vi "MPU_Stick_main.vi"() -> ()   [LabVIEW 2017]
uses:
  Controls/IMU_Accelerometer_Full_Scale_Values.ctl
  Controls/IMU_Accelerometer_Bandwidth.ctl
  Controls/IMU_Gyroscope_Full_Scale_Values.ctl
  Controls/IMU_Gyroscope_Bandwidth.ctl
  Controls/LED_config.ctl
  Controls/Motion_Detection_Threshold_Type.ctl
  Controls/MPU_Stick_Plotter_Parameters.ctl
  Controls/MPU_Stick_Globals.ctl
  Controls/IMU_Configuration_References.ctl
  Controls/MP_Comp_Filter_Constants_References.ctl
  Controls/MD_Threshold_References.ctl
  Controls/MD_Type_References.ctl
  Controls/LED_Configuration_References.ctl
  Controls/Primary_References.ctl
  Controls/MPU_Stick_Queues.ctl
  Controls/MPU_Stick_Queue_Element.ctl
  Controls/MPU_Stick_Queue_Commands.ctl
  Classes/ADCP.lvclass
panel:
  in  "Tab Control":enum32{"Configurations", "Data and plot"}(tab)
  in  "Save all config.":bool
  in  "Write all config.":bool
  in  "Read all config.":bool
  in  "Set pitch filter constant":bool
  in  "Get pitch filter constant":bool
  in  "Set roll filter constant":bool
  in  "Get roll filter constant":bool
  in  "Pitch filter constant":dbl
  in  "Roll filter constant":dbl
  in  "Get all Motion detection threshold configurations":bool
  in  "Set all Motion detection threshold configurations":bool
  in  "Set yaw threshold (upper)":bool
  in  "Get yaw threshold (upper)":bool
  in  "Set yaw threshold (lower)":bool
  in  "Get yaw threshold (lower)":bool
  in  "Set pitch threshold (upper)":bool
  in  "Get pitch threshold (upper)":bool
  in  "Set pitch threshold (lower)":bool
  in  "Get pitch threshold (lower)":bool
  in  "Set roll threshold (upper)":bool
  in  "Get roll threshold (upper)":bool
  in  "Set roll threshold (lower)":bool
  in  "Get roll threshold (lower)":bool
  in  "Yaw threshold (U)":dbl
  in  "Yaw threshold (L)":dbl
  in  "Pitch threshold (U)":dbl
  in  "Pitch. threshold (L)":dbl
  in  "Roll threshold (U)":dbl
  in  "Roll threshold (L)":dbl
  in  "Set Z gyro threshold (upper)":bool
  in  "Get Z gyro threshold (upper)":bool
  in  "Set Z gyro threshold (lower)":bool
  in  "Get Z gyro threshold (lower)":bool
  in  "Set Y gyro threshold (upper)":bool
  in  "Get Y gyro threshold (upper)":bool
  in  "Set Y gyro threshold (lower)":bool
  in  "Get Y gyro threshold (lower)":bool
  in  "Set X gyro threshold (upper)":bool
  in  "Get X gyro threshold (upper)":bool
  in  "Set X gyro threshold (lower)":bool
  in  "Get X gyro threshold (lower)":bool
  in  "Z gyro. threshold (U)":dbl
  in  "Z gyro. threshold (L)":dbl
  in  "Y gyro. threshold (U)":dbl
  in  "Y gyro. threshold (L)":dbl
  in  "X gyro. threshold (U)":dbl
  in  "X gyro. threshold (L)":dbl
  in  "Set Z accel threshold (upper)":bool
  in  "Get Z accel threshold (upper)":bool
  in  "Set Z accel threshold (lower)":bool
  in  "Get Z accel threshold (lower)":bool
  in  "Set Y accel threshold (upper)":bool
  in  "Get Y accel threshold (upper)":bool
  in  "Set Y accel threshold (lower)":bool
  in  "Get Y accel threshold (lower)":bool
  in  "Set X accel threshold (upper)":bool
  in  "Get X accel threshold (upper)":bool
  in  "Set X accel threshold (lower)":bool
  in  "Get X accel threshold (lower)":bool
  in  "Z accel. threshold (U)":dbl
  in  "Z accel. threshold (L)":dbl
  in  "Y accel. threshold (U)":dbl
  in  "Y accel. threshold (L)":dbl
  in  "X accel. threshold (U)":dbl
  in  "X accel. threshold (L)":dbl
  in  "Set all Motion detection type configurations":bool
  in  "Get all Motion detection type configurations":bool
  in  "Set yaw threshold type":bool
  in  "Get yaw threshold type":bool
  in  "Set pitch threshold type":bool
  in  "Get pitch threshold type":bool
  in  "Set roll threshold type":bool
  in  "Get roll threshold type":bool
  in  "Set Z gyroscope threshold type":bool
  in  "Get Z gyroscope threshold type":bool
  in  "Set Y gyroscope threshold type":bool
  in  "Get Y gyroscope threshold type":bool
  in  "Set X gyroscope threshold type":bool
  in  "Get X gyroscope threshold type":bool
  in  "Set Z accel threshold type":bool
  in  "Get Z accel threshold type":bool
  in  "Set Y accel threshold type":bool
  in  "Get Y accel threshold type":bool
  in  "Yaw threshold type":T1
  in  "Pitch threshold type":T1
  in  "Roll threshold type":T1
  in  "Z gyro threshold type":T1
  in  "Y gyro threshold type":T1
  in  "X gyro threshold type":T1
  in  "Z accel threshold type":T1
  in  "Y accel threshold type":T1
  in  "IMU Accelerometer F.S. value":T2
  in  "IMU Accelerometer bandwidth":T3
  in  "IMU Gyroscope F.S. value":T4
  in  "IMU Gyroscope bandwidth":T5
  in  "Calibration interval (ms)":u16
  in  "Calibration point count":u16
  in  "Sampling frequency (Hz)":u16
  in  "Set Accelerometer F.S. Value":bool
  in  "Get Accelerometer F.S. Value":bool
  in  "Set Accelerometer bandwidth":bool
  in  "Get Accelerometer bandwidth":bool
  in  "Set Gyroscope F.S. Value":bool
  in  "Get Gyroscope F.S. Value":bool
  in  "Set Gyroscope bandwidth":bool
  in  "Get Gyroscope bandwidth":bool
  in  "Set calibration interval":bool
  in  "Get calibration interval":bool
  in  "Set calibration point count":bool
  in  "Get calibration point count":bool
  in  "Set sampling frequency":bool
  in  "Get sampling frequency":bool
  in  "Set all IMU configurations":bool
  in  "Get all IMU configurations":bool
  in  "COM Port":refnum<visa-resource-name>="COM13"
  in  "Baud Rate":u32=38400
  in  "Connect Device":bool
  in  "LED1 Configuration":T6
  in  "LED2 Configuration":T6
  in  "LED3 Configuration":T6
  in  "Set LED1 configuration":bool
  in  "Get LED1 configuration":bool
  in  "Set LED2 configuration":bool
  in  "Get LED2 configuration":bool
  in  "Set LED3 configuration":bool
  in  "Get LED3 configuration":bool
  in  "Set all LED configurations":bool
  in  "Get all LED configurations":bool
  in  "X accel threshold type":T1
  in  "Set X accel threshold type":bool
  in  "Get X accel threshold type":bool
  out "Progress Bar":u8(slide) caption="No operation" scale=0.0..100.0
  out "Parameter name":string
  out "Plot time (ms)":dbl
  out "Plot value":dbl
  in  "Get Range & Offset":bool
  in  "Set Range & Offset":bool
  in  "Offset":dbl min=-100000.0 max=100000.0 step=0.1
  in  "Range":dbl min=0.0 max=100000.0 step=0.1
  in  "Exit Application":bool
  in  "Time (ms)":dbl
  in  "Value (Units)":dbl
  in  "Graph / 3D view tab control":enum32{"3D View", "Graph"}(tab)=enum."Graph"
  out "3D View Image":refnum<vi>(3d-picture)
  out "Plot":cluster{"Values":dbl[], "Time (ms)":dbl[]}[](graph)
  in  "MP Reset":bool
  in  "Calibrate IMU":bool
  out "Plot Parameter List":string[](array[string])
  in  "Remove Parameter from Plot":bool
  in  "Add Parameter to Plot":bool
  in  "Parameter to monitor":T7
  out "Yaw MD O/P":bool
  out "Pitch MD O/P":bool
  out "Roll MD O/P":bool
  out "Z gyro MD O/P":bool
  out "Y gyro MD O/P":bool
  out "X gyro MD O/P":bool
  out "Z accel MD O/P":bool
  out "Y accel MD O/P":bool
  out "X accel MD O/P":bool
  out "Roll angle (filter) (degrees)":dbl
  out "Pitch angle (filter) (degrees)":dbl
  out "Yaw angle (filter) (degrees)":dbl
  out "Roll angle (gyro) (degrees)":dbl
  out "Pitch angle (gyro) (degrees)":dbl
  out "Yaw angle (gyro) (degrees)":dbl
  out "Z accelerometer reading (G)":dbl
  out "Y accelerometer reading (G)":dbl
  out "X accelerometer reading (G)":dbl
  out "X gyroscope reading (DPS)":dbl
  out "Y gyroscope reading (DPS)":dbl
  out "Z gyroscope reading (DPS)":dbl
  out "Roll angle (accel) (degrees)":dbl
  out "Pitch angle (accel) (degrees)":dbl
  out "Yaw angle (accel) (degrees)":dbl
  # "LED CONFIGURATIONS"
  # "MOTION PROCESSING DETECTION CONFIGURATIONS"
  # "IMU CONFIGURATIONS"
  # "COMPLEMENTARY FILTER CONSTANTS"
  # "MOTION PROCESSED THRESHOLD CONFIGURATIONS"
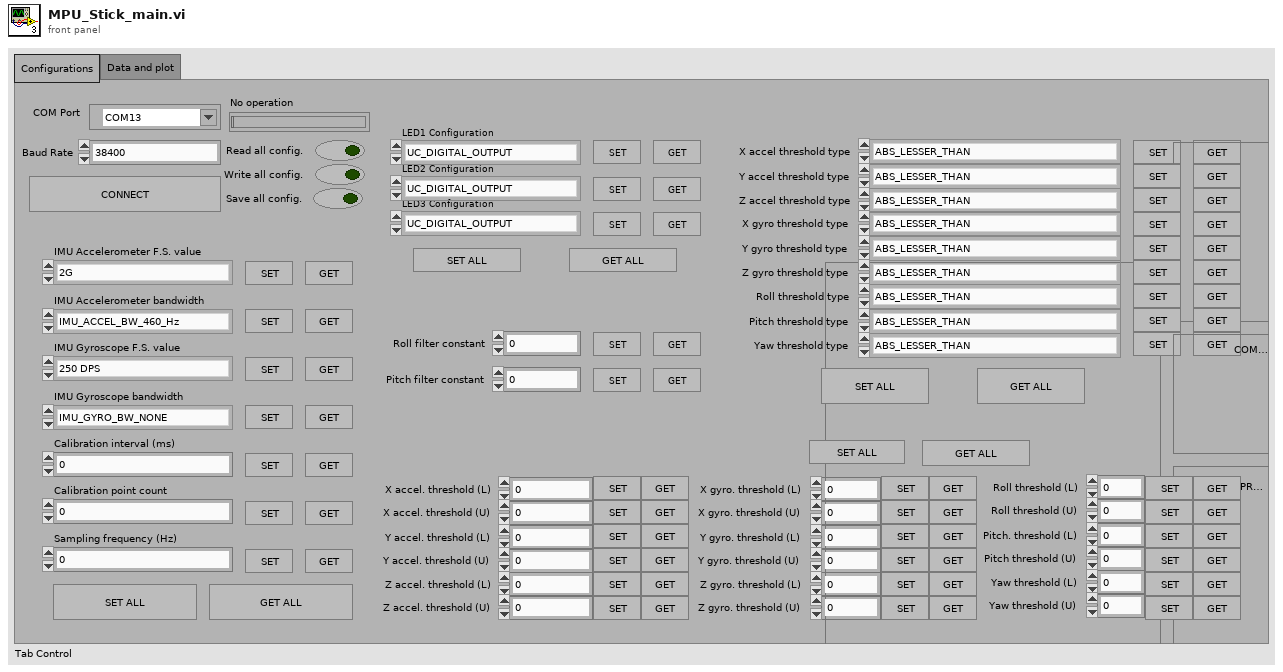
[diagram p1: front panel]
types:
  T1 = typedef "Motion_Detection_Threshold_Type.ctl" = enum16{"ABS_LESSER_THAN", "ABS_GREATER_THAN", "LESSER_THAN", "GREATER_THAN", "WINDOWED_MODE_WITHIN_BOUNDS", "WINDOWED_MODE_OUTSIDE_BOUNDS"}
  T2 = typedef "IMU_Accelerometer_Full_Scale_Values.ctl" = enum16{"2G", "4G", "8G", "16G"}
  T3 = typedef "IMU_Accelerometer_Bandwidth.ctl" = enum16{"IMU_ACCEL_BW_460_Hz", "IMU_ACCEL_BW_184_Hz", "IMU_ACCEL_BW_92_Hz", "IMU_ACCEL_BW_41_Hz", "IMU_ACCEL_BW_20_Hz", "IMU_ACCEL_BW_10_Hz", "IMU_ACCEL_BW_5_Hz"}
  T4 = typedef "IMU_Gyroscope_Full_Scale_Values.ctl" = enum16{"250 DPS", "500 DPS", "1000 DPS", "2000 DPS"}
  T5 = typedef "IMU_Gyroscope_Bandwidth.ctl" = enum16{"IMU_GYRO_BW_NONE", "IMU_GYRO_BW_184_Hz", "IMU_GYRO_BW_92_Hz", "IMU_GYRO_BW_41_Hz", "IMU_GYRO_BW_20_Hz", "IMU_GYRO_BW_10_Hz", "IMU_GYRO_BW_5_Hz"}
  T6 = typedef "LED_config.ctl" = enum16{"UC_DIGITAL_OUTPUT", "X_ACCEL_PWM", "Y_ACCEL_PWM", "Z_ACCEL_PWM", "X_ACCEL_MD_OUTPUT", "Y_ACCEL_MD_OUTPUT", "Z_ACCEL_MD_OUTPUT", "X_GYRO_PWM", "Y_GYRO_PWM", "Z_GYRO_PWM", "X_GYRO_MD_OUTPUT", "Y_GYRO_MD_OUTPUT", "Z_GYRO_MD_OUTPUT", "ROLL_PWM_OUTPUT", "PITCH_PWM_OUTPUT", "YAW_PWM_OUTPUT", "ROLL_MD_OUTPUT", "PITCH_MD_OUTPUT", "YAW_MD_OUTPUT", "UC_PWM_OUTPUT"}
  T7 = typedef "MPU_Stick_Plotter_Parameters.ctl" = enum16{"ACCEL_X", "ACCEL_Y", "ACCEL_Z", "GYRO_X", "GYRO_Y", "GYRO_Z", "ROLL_ACCEL", "ROLL_GYRO", "ROLL_COMP_FILTER", "PITCH_ACCEL", "PITCH_GYRO", "PITCH_COMP_FILTER", "YAW_ACCEL", "YAW_GYRO", "YAW_COMP_FILTER"}
  T8 = typedef "MPU_Stick_Globals.ctl" = cluster{"IMU_configuration_references":T9, "MP_Comp_Filter_Constants_References":T10, "MD_Threshold_References":T11, "MD_Type_References":T12, "LED_Configuration_References":T13, "Primary_references":T14, "MPU_Stick_Queues":T15, "ADCP":refnum<vi>}
  T9 = typedef "IMU_Configuration_References.ctl" = cluster{"Get all IMU configurations":refnum<vi>, "Set all IMU configurations":refnum<vi>, "Get sampling frequency":refnum<vi>, "Set sampling frequency":refnum<vi>, "Get calibration point count":refnum<vi>, "Set calibration point count":refnum<vi>, "Get calibration interval":refnum<vi>, "Set calibration interval":refnum<vi>, "Get Gyroscope bandwidth":refnum<vi>, "Set Gyroscope bandwidth":refnum<vi>, "Get Gyroscope F.S. Value":refnum<vi>, "Set Gyroscope F.S. Value":refnum<vi>, "Get Accelerometer bandwidth":refnum<vi>, "Set Accelerometer bandwidth":refnum<vi>, "Get Accelerometer F.S. Value":refnum<vi>, "Set Accelerometer F.S. Value":refnum<vi>, "Sampling frequency (Hz)":refnum<vi>, "Calibration point count":refnum<vi>, "Calibration interval (ms)":refnum<vi>, "IMU Gyroscope bandwidth":refnum<vi>, "IMU Gyroscope F.S. value":refnum<vi>, "IMU Accelerometer bandwidth":refnum<vi>, "IMU Accelerometer F.S. value":refnum<vi>}
  T10 = typedef "MP_Comp_Filter_Constants_References.ctl" = cluster{"Set pitch filter constant":refnum<vi>, "Get pitch filter constant":refnum<vi>, "Set roll filter constant":refnum<vi>, "Get roll filter constant":refnum<vi>, "Pitch filter constant":refnum<vi>, "Roll filter constant":refnum<vi>}
  T11 = typedef "MD_Threshold_References.ctl" = cluster{"Yaw threshold (U)":refnum<vi>, "Yaw threshold (L)":refnum<vi>, "Pitch threshold (U)":refnum<vi>, "Pitch. threshold (L)":refnum<vi>, "Roll threshold (U)":refnum<vi>, "Roll threshold (L)":refnum<vi>, "Z gyro. threshold (U)":refnum<vi>, "Z gyro. threshold (L)":refnum<vi>, "Y gyro. threshold (U)":refnum<vi>, "Y gyro. threshold (L)":refnum<vi>, "X gyro. threshold (U)":refnum<vi>, "X gyro. threshold (L)":refnum<vi>, "Z accel. threshold (U)":refnum<vi>, "Z accel. threshold (L)":refnum<vi>, "Y accel. threshold (U)":refnum<vi>, "Y accel. threshold (L)":refnum<vi>, "X accel. threshold (U)":refnum<vi>, "X accel. threshold (L)":refnum<vi>, "Set all Motion detection threshold configurations":refnum<vi>, "Get yaw threshold (upper)":refnum<vi>, "Get yaw threshold (lower)":refnum<vi>, "Get pitch threshold (upper)":refnum<vi>, "Get pitch threshold (lower)":refnum<vi>, "Get roll threshold (upper)":refnum<vi>, "Get roll threshold (lower)":refnum<vi>, "Get Z gyro threshold (upper)":refnum<vi>, "Get Z gyro threshold (lower)":refnum<vi>, "Get Y gyro threshold (upper)":refnum<vi>, "Get Y gyro threshold (lower)":refnum<vi>, "Get X gyro threshold (upper)":refnum<vi>, "Get X gyro threshold (lower)":refnum<vi>, "Get Z accel threshold (upper)":refnum<vi>, "Get Z accel threshold (lower)":refnum<vi>, "Get Y accel threshold (upper)":refnum<vi>, "Get Y accel threshold (lower)":refnum<vi>, "Get X accel threshold (upper)":refnum<vi>, "Get X accel threshold (lower)":refnum<vi>, "Get all Motion detection threshold configurations":refnum<vi>, "Set yaw threshold (upper)":refnum<vi>, "Set yaw threshold (lower)":refnum<vi>, "Set pitch threshold (upper)":refnum<vi>, "Set pitch threshold (lower)":refnum<vi>, "Set roll threshold (upper)":refnum<vi>, "Set roll threshold (lower)":refnum<vi>, "Set Z gyro threshold (upper)":refnum<vi>, "Set Z gyro threshold (lower)":refnum<vi>, "Set Y gyro threshold (upper)":refnum<vi>, "Set Y gyro threshold (lower)":refnum<vi>, "Set X gyro threshold (upper)":refnum<vi>, "Set X gyro threshold (lower)":refnum<vi>, "Set Z accel threshold (upper)":refnum<vi>, "Set Z accel threshold (lower)":refnum<vi>, "Set Y accel threshold (upper)":refnum<vi>, "Set Y accel threshold (lower)":refnum<vi>, "Set X accel threshold (upper)":refnum<vi>, "Set X accel threshold (lower)":refnum<vi>}
  T12 = typedef "MD_Type_References.ctl" = cluster{"Yaw threshold type":refnum<vi>, "Pitch threshold type":refnum<vi>, "Roll threshold type":refnum<vi>, "Z gyro threshold type":refnum<vi>, "Y gyro threshold type":refnum<vi>, "X gyro threshold type":refnum<vi>, "Z accel threshold type":refnum<vi>, "Y accel threshold type":refnum<vi>, "X accel threshold type":refnum<vi>, "Set all Motion detection type configurations":refnum<vi>, "Get all Motion detection type configurations":refnum<vi>, "Set yaw threshold type":refnum<vi>, "Get yaw threshold type":refnum<vi>, "Set pitch threshold type":refnum<vi>, "Get pitch threshold type":refnum<vi>, "Set roll threshold type":refnum<vi>, "Get roll threshold type":refnum<vi>, "Set Z gyroscope threshold type":refnum<vi>, "Get Z gyroscope threshold type":refnum<vi>, "Set Y gyroscope threshold type":refnum<vi>, "Get Y gyroscope threshold type":refnum<vi>, "Set X gyroscope threshold type":refnum<vi>, "Get X gyroscope threshold type":refnum<vi>, "Set Z accel threshold type":refnum<vi>, "Get Z accel threshold type":refnum<vi>, "Set Y accel threshold type":refnum<vi>, "Get Y accel threshold type":refnum<vi>, "Get X accel threshold type":refnum<vi>, "Set X accel threshold type":refnum<vi>}
  T13 = typedef "LED_Configuration_References.ctl" = cluster{"Get all LED configurations":refnum<vi>, "Set all LED configurations":refnum<vi>, "Get LED3 configuration":refnum<vi>, "Set LED3 configuration":refnum<vi>, "Get LED2 configuration":refnum<vi>, "Set LED2 configuration":refnum<vi>, "Get LED1 configuration":refnum<vi>, "Set LED1 configuration":refnum<vi>, "LED3 Configuration":refnum<vi>, "LED2 Configuration":refnum<vi>, "LED1 Configuration":refnum<vi>}
  T14 = typedef "Primary_References.ctl" = cluster{"3D View Image":refnum<vi>, "Plot":refnum<vi>, "Graph / 3D view tab control":refnum<vi>, "MP Reset":refnum<vi>, "Calibrate IMU":refnum<vi>, "Plot Parameter List":refnum<vi>, "Remove Parameter from Plot":refnum<vi>, "Add Parameter to Plot":refnum<vi>, "Parameter to monitor":refnum<vi>, "Yaw motion detection output":refnum<vi>, "Pitch motion detection output":refnum<vi>, "Roll motion detection output":refnum<vi>, "Z gyro motion detection output":refnum<vi>, "Y gyro motion detection output":refnum<vi>, "X gyro motion detection output":refnum<vi>, "Z accel motion detection output":refnum<vi>, "Y accel motion detection output":refnum<vi>, "X accel motion detection output":refnum<vi>, "Yaw angle (filter) (degrees)":refnum<vi>, "Pitch angle (filter) (degrees)":refnum<vi>, "Roll angle (filter) (degrees)":refnum<vi>, "Yaw angle (gyro) (degrees)":refnum<vi>, "Pitch angle (gyro) (degrees)":refnum<vi>, "Roll angle (gyro) (degrees)":refnum<vi>, "Yaw angle (accel) (degrees)":refnum<vi>, "Pitch angle (accel) (degrees)":refnum<vi>, "Roll angle (accel) (degrees)":refnum<vi>, "Z gyroscope reading (DPS)":refnum<vi>, "Y gyroscope reading (DPS)":refnum<vi>, "X gyroscope reading (DPS)":refnum<vi>, "Z accelerometer reading (G)":refnum<vi>, "Y accelerometer reading (G)":refnum<vi>, "X accelerometer reading (G)":refnum<vi>, "Save all config.":refnum<vi>, "Write all config.":refnum<vi>, "Read all config.":refnum<vi>, "Tab Control":refnum<vi>, "Baud Rate":refnum<vi>, "COM Port":refnum<vi>, "Time (ms)":refnum<vi>, "Value (Units)":refnum<vi>, "Exit Application":refnum<vi>, "Connect Device":refnum<vi>, "Progress Bar":refnum<vi>, "Get Range & Offset":refnum<vi>, "Range":refnum<vi>, "Offset":refnum<vi>, "Set Range & Offset":refnum<vi>, "Parameter name":refnum<vi>, "Plot time (ms)":refnum<vi>, "Plot value":refnum<vi>}
  T15 = typedef "MPU_Stick_Queues.ctl" = cluster{"UI Event Handler":refnum<queue>, "3D View Updater":refnum<queue>, "Plot Updater":refnum<queue>, "Serial Port Reader":refnum<queue>, "UI Indicators Updater":refnum<queue>}
diagram:
  n1 = control-ref of="This VI"() -> (w3:refnum<vi>)
  n2 = invoke class="VI" method="Default Vals.Reinit All"(reference=w3, error in=errorcluster {"status"=FALSE, "code"=0, "source"=""} ("error constant")) -> (error out=w4:errorcluster)  [unwired: 1 in, 2 out]
  n3 = flat-sequence {
    tunnel: w4 -> [w60]
    tunnel: [w60] -> w34
    tunnel: [w35] -> w29
    frame #0 {
      # "IMU Configuration Controls"
      n4 = control-ref of="Get Accelerometer F.S. Value"() -> (w44:refnum<vi>)
      n5 = control-ref of="Set Accelerometer F.S. Value"() -> (w43:refnum<vi>)
      n6 = control-ref of="Get all IMU configurations"() -> (w58:refnum<vi>)
      n7 = control-ref of="Get sampling frequency"() -> (w56:refnum<vi>)
      n8 = control-ref of="Set sampling frequency"() -> (w55:refnum<vi>)
      n9 = control-ref of="Set calibration point count"() -> (w53:refnum<vi>)
      n10 = control-ref of="Get calibration interval"() -> (w52:refnum<vi>)
      n11 = control-ref of="Set Gyroscope bandwidth"() -> (w49:refnum<vi>)
      n12 = control-ref of="Get Gyroscope F.S. Value"() -> (w48:refnum<vi>)
      n13 = control-ref of="Get Accelerometer bandwidth"() -> (w46:refnum<vi>)
      n14 = control-ref of="Set Accelerometer bandwidth"() -> (w45:refnum<vi>)
      n15 = control-ref of="Set all IMU configurations"() -> (w57:refnum<vi>)
      n16 = control-ref of="Get calibration point count"() -> (w54:refnum<vi>)
      n17 = control-ref of="Set calibration interval"() -> (w51:refnum<vi>)
      n18 = control-ref of="Get Gyroscope bandwidth"() -> (w50:refnum<vi>)
      n19 = control-ref of="Set Gyroscope F.S. Value"() -> (w47:refnum<vi>)
      n20 = control-ref of="Calibration interval (ms)"() -> (w40:refnum<vi>)
      n21 = control-ref of="Sampling frequency (Hz)"() -> (w42:refnum<vi>)
      n22 = control-ref of="Calibration point count"() -> (w41:refnum<vi>)
      n23 = control-ref of="IMU Gyroscope bandwidth"() -> (w39:refnum<vi>)
      n24 = control-ref of="IMU Gyroscope F.S. value"() -> (w38:refnum<vi>)
      n25 = control-ref of="IMU Accelerometer bandwidth"() -> (w37:refnum<vi>)
      n26 = control-ref of="IMU Accelerometer F.S. value"() -> (w36:refnum<vi>)
      n27 = Bundle By Name(cluster=T9 {"Get all IMU configurations"=refnum, "Set all IMU configurations"=refnum, "Get sampling frequency"=refnum, "Set sampling frequency"=refnum, "Get calibration point count"=refnum, "Set calibration point count"=refnum, "Get calibration interval"=refnum, "Set calibration interval"=refnum, "Get Gyroscope bandwidth"=refnum, "Set Gyroscope bandwidth"=refnum, "Get Gyroscope F.S. Value"=refnum, "Set Gyroscope F.S. Value"=refnum, "Get Accelerometer bandwidth"=refnum, "Set Accelerometer bandwidth"=refnum, "Get Accelerometer F.S. Value"=refnum, "Set Accelerometer F.S. Value"=refnum, "Sampling frequency (Hz)"=refnum, "Calibration point count"=refnum, "Calibration interval (ms)"=refnum, "IMU Gyroscope bandwidth"=refnum, "IMU Gyroscope F.S. value"=refnum, "IMU Accelerometer bandwidth"=refnum, "IMU Accelerometer F.S. value"=refnum} ("IMU configuration references"), "Get all IMU configurations"=w58, "Set all IMU configurations"=w57, "Get sampling frequency"=w56, "Set sampling frequency"=w55, "Get calibration point count"=w54, "Set calibration point count"=w53, "Get calibration interval"=w52, "Set calibration interval"=w51, "Get Gyroscope bandwidth"=w50, "Set Gyroscope bandwidth"=w49, "Get Gyroscope F.S. Value"=w48, "Set Gyroscope F.S. Value"=w47, "Get Accelerometer bandwidth"=w46, "Set Accelerometer bandwidth"=w45, "Get Accelerometer F.S. Value"=w44, "Set Accelerometer F.S. Value"=w43, "Sampling frequency (Hz)"=w42, "Calibration point count"=w41, "Calibration interval (ms)"=w40, "IMU Gyroscope bandwidth"=w39, "IMU Gyroscope F.S. value"=w38, "IMU Accelerometer bandwidth"=w37, "IMU Accelerometer F.S. value"=w36) -> (w35:T9)
    }
  }
  n28 = flat-sequence {
    tunnel: w34 -> [w115]
    tunnel: [w115] -> w33
    tunnel: w29 -> [w73]
    tunnel: [w73] -> w28
    tunnel: [w72] -> w24
    frame #0 {
      # "UI primary controls & indicators"
      n29 = control-ref of="MP Reset"() -> (w110:refnum<vi>)
      n30 = control-ref of="Graph / 3D view tab control"() -> (w111:refnum<vi>)
      n31 = control-ref of="Calibrate IMU"() -> (w109:refnum<vi>)
      n32 = control-ref of="3D View Image"() -> (w113:refnum<vi>)
      n33 = control-ref of="Plot"() -> (w112:refnum<vi>)
      n34 = control-ref of="X accel MD O/P"() -> (w96:refnum<vi>)
      n35 = control-ref of="Y accel MD O/P"() -> (w97:refnum<vi>)
      n36 = control-ref of="Plot Parameter List"() -> (w108:refnum<vi>)
      n37 = control-ref of="Remove Parameter from Plot"() -> (w107:refnum<vi>)
      n38 = control-ref of="Add Parameter to Plot"() -> (w106:refnum<vi>)
      n39 = control-ref of="Parameter to monitor"() -> (w105:refnum<vi>)
      n40 = control-ref of="X gyro MD O/P"() -> (w99:refnum<vi>)
      n41 = control-ref of="Z accel MD O/P"() -> (w98:refnum<vi>)
      n42 = control-ref of="Yaw angle (filter) (degrees)"() -> (w95:refnum<vi>)
      n43 = control-ref of="Yaw MD O/P"() -> (w104:refnum<vi>)
      n44 = control-ref of="Pitch MD O/P"() -> (w103:refnum<vi>)
      n45 = control-ref of="Roll MD O/P"() -> (w102:refnum<vi>)
      n46 = control-ref of="Z gyro MD O/P"() -> (w101:refnum<vi>)
      n47 = control-ref of="Y gyro MD O/P"() -> (w100:refnum<vi>)
      n48 = control-ref of="Pitch angle (filter) (degrees)"() -> (w94:refnum<vi>)
      n49 = control-ref of="COM Port"() -> (w74:refnum<vi>)
      n50 = control-ref of="Roll angle (filter) (degrees)"() -> (w93:refnum<vi>)
      n51 = control-ref of="Save all config."() -> (w80:refnum<vi>)
      n52 = control-ref of="Write all config."() -> (w79:refnum<vi>)
      n53 = control-ref of="Tab Control"() -> (w77:refnum<vi>)
      n54 = control-ref of="Connect Device"() -> (w76:refnum<vi>)
      n55 = control-ref of="Baud Rate"() -> (w75:refnum<vi>)
      n56 = control-ref of="Pitch angle (gyro) (degrees)"() -> (w91:refnum<vi>)
      n57 = control-ref of="X gyroscope reading (DPS)"() -> (w84:refnum<vi>)
      n58 = control-ref of="Read all config."() -> (w78:refnum<vi>)
      n59 = control-ref of="Yaw angle (gyro) (degrees)"() -> (w92:refnum<vi>)
      n60 = control-ref of="Roll angle (gyro) (degrees)"() -> (w90:refnum<vi>)
      n61 = control-ref of="Yaw angle (accel) (degrees)"() -> (w89:refnum<vi>)
      n62 = control-ref of="Roll angle (accel) (degrees)"() -> (w87:refnum<vi>)
      n63 = control-ref of="Z gyroscope reading (DPS)"() -> (w86:refnum<vi>)
      n64 = control-ref of="Y gyroscope reading (DPS)"() -> (w85:refnum<vi>)
      n65 = control-ref of="Time (ms)"() -> (w71:refnum<vi>)
      n66 = control-ref of="Value (Units)"() -> (w70:refnum<vi>)
      n67 = control-ref of="Exit Application"() -> (w69:refnum<vi>)
      n68 = control-ref of="Progress Bar"() -> (w68:refnum<vi>)
      n69 = control-ref of="Pitch angle (accel) (degrees)"() -> (w88:refnum<vi>)
      n70 = control-ref of="Z accelerometer reading (G)"() -> (w83:refnum<vi>)
      n71 = control-ref of="Y accelerometer reading (G)"() -> (w82:refnum<vi>)
      n72 = control-ref of="X accelerometer reading (G)"() -> (w81:refnum<vi>)
      n73 = control-ref of="Get Range & Offset"() -> (w67:refnum<vi>)
      n74 = control-ref of="Range"() -> (w66:refnum<vi>)
      n75 = control-ref of="Offset"() -> (w65:refnum<vi>)
      n76 = control-ref of="Set Range & Offset"() -> (w64:refnum<vi>)
      n77 = control-ref of="Parameter name"() -> (w63:refnum<vi>)
      n78 = control-ref of="Plot time (ms)"() -> (w62:refnum<vi>)
      n79 = control-ref of="Plot value"() -> (w61:refnum<vi>)
      n80 = Bundle By Name(cluster=T14 {"3D View Image"=refnum, "Plot"=refnum, "Graph / 3D view tab control"=refnum, "MP Reset"=refnum, "Calibrate IMU"=refnum, "Plot Parameter List"=refnum, "Remove Parameter from Plot"=refnum, "Add Parameter to Plot"=refnum, "Parameter to monitor"=refnum, "Yaw motion detection output"=refnum, "Pitch motion detection output"=refnum, "Roll motion detection output"=refnum, "Z gyro motion detection output"=refnum, "Y gyro motion detection output"=refnum, "X gyro motion detection output"=refnum, "Z accel motion detection output"=refnum, "Y accel motion detection output"=refnum, "X accel motion detection output"=refnum, "Yaw angle (filter) (degrees)"=refnum, "Pitch angle (filter) (degrees)"=refnum, "Roll angle (filter) (degrees)"=refnum, "Yaw angle (gyro) (degrees)"=refnum, "Pitch angle (gyro) (degrees)"=refnum, "Roll angle (gyro) (degrees)"=refnum, "Yaw angle (accel) (degrees)"=refnum, "Pitch angle (accel) (degrees)"=refnum, "Roll angle (accel) (degrees)"=refnum, "Z gyroscope reading (DPS)"=refnum, "Y gyroscope reading (DPS)"=refnum, "X gyroscope reading (DPS)"=refnum, "Z accelerometer reading (G)"=refnum, "Y accelerometer reading (G)"=refnum, "X accelerometer reading (G)"=refnum, "Save all config."=refnum, "Write all config."=refnum, "Read all config."=refnum, "Tab Control"=refnum, "Baud Rate"=refnum, "COM Port"=refnum, "Time (ms)"=refnum, "Value (Units)"=refnum, "Exit Application"=refnum, "Connect Device"=refnum, "Progress Bar"=refnum, "Get Range & Offset"=refnum, "Range"=refnum, "Offset"=refnum, "Set Range & Offset"=refnum, "Parameter name"=refnum, "Plot time (ms)"=refnum, "Plot value"=refnum}, "3D View Image"=w113, "Plot"=w112, "Graph / 3D view tab control"=w111, "MP Reset"=w110, "Calibrate IMU"=w109, "Plot Parameter List"=w108, "Remove Parameter from Plot"=w107, "Add Parameter to Plot"=w106, "Parameter to monitor"=w105, "Yaw motion detection output"=w104, "Pitch motion detection output"=w103, "Roll motion detection output"=w102, "Z gyro motion detection output"=w101, "Y gyro motion detection output"=w100, "X gyro motion detection output"=w99, "Z accel motion detection output"=w98, "Y accel motion detection output"=w97, "X accel motion detection output"=w96, "Yaw angle (filter) (degrees)"=w95, "Pitch angle (filter) (degrees)"=w94, "Roll angle (filter) (degrees)"=w93, "Yaw angle (gyro) (degrees)"=w92, "Pitch angle (gyro) (degrees)"=w91, "Roll angle (gyro) (degrees)"=w90, "Yaw angle (accel) (degrees)"=w89, "Pitch angle (accel) (degrees)"=w88, "Roll angle (accel) (degrees)"=w87, "Z gyroscope reading (DPS)"=w86, "Y gyroscope reading (DPS)"=w85, "X gyroscope reading (DPS)"=w84, "Z accelerometer reading (G)"=w83, "Y accelerometer reading (G)"=w82, "X accelerometer reading (G)"=w81, "Save all config."=w80, "Write all config."=w79, "Read all config."=w78, "Tab Control"=w77, "Connect Device"=w76, "Baud Rate"=w75, "COM Port"=w74, "Time (ms)"=w71, "Value (Units)"=w70, "Exit Application"=w69, "Progress Bar"=w68, "Get Range & Offset"=w67, "Range"=w66, "Offset"=w65, "Set Range & Offset"=w64, "Parameter name"=w63, "Plot time (ms)"=w62, "Plot value"=w61) -> (w72:T14)
    }
  }
  n81 = flat-sequence {
    tunnel: w33 -> [w131]
    tunnel: [w131] -> w32
    tunnel: w28 -> [w118]
    tunnel: [w118] -> w27
    tunnel: w24 -> [w117]
    tunnel: [w117] -> w23
    tunnel: [w116] -> w20
    frame #0 {
      # "LED configurations"
      n82 = control-ref of="Get all LED configurations"() -> (w129:refnum<vi>)
      n83 = control-ref of="Set all LED configurations"() -> (w128:refnum<vi>)
      n84 = control-ref of="Get LED3 configuration"() -> (w127:refnum<vi>)
      n85 = control-ref of="Set LED3 configuration"() -> (w126:refnum<vi>)
      n86 = control-ref of="Get LED2 configuration"() -> (w125:refnum<vi>)
      n87 = control-ref of="Set LED2 configuration"() -> (w124:refnum<vi>)
      n88 = control-ref of="Get LED1 configuration"() -> (w123:refnum<vi>)
      n89 = control-ref of="Set LED1 configuration"() -> (w122:refnum<vi>)
      n90 = control-ref of="LED3 Configuration"() -> (w121:refnum<vi>)
      n91 = control-ref of="LED2 Configuration"() -> (w120:refnum<vi>)
      n92 = control-ref of="LED1 Configuration"() -> (w119:refnum<vi>)
      n93 = Bundle By Name(cluster=T13 {"Get all LED configurations"=refnum, "Set all LED configurations"=refnum, "Get LED3 configuration"=refnum, "Set LED3 configuration"=refnum, "Get LED2 configuration"=refnum, "Set LED2 configuration"=refnum, "Get LED1 configuration"=refnum, "Set LED1 configuration"=refnum, "LED3 Configuration"=refnum, "LED2 Configuration"=refnum, "LED1 Configuration"=refnum}, "Get all LED configurations"=w129, "Set all LED configurations"=w128, "Get LED3 configuration"=w127, "Set LED3 configuration"=w126, "Get LED2 configuration"=w125, "Set LED2 configuration"=w124, "Get LED1 configuration"=w123, "Set LED1 configuration"=w122, "LED3 Configuration"=w121, "LED2 Configuration"=w120, "LED1 Configuration"=w119) -> (w116:T13)
    }
  }
  n94 = flat-sequence {
    tunnel: w32 -> [w167]
    tunnel: [w167] -> w31
    tunnel: w27 -> [w135]
    tunnel: [w135] -> w26
    tunnel: w23 -> [w134]
    tunnel: [w134] -> w22
    tunnel: w20 -> [w133]
    tunnel: [w133] -> w19
    tunnel: [w132] -> w17
    frame #0 {
      # "Motion detection threshold types"
      n95 = control-ref of="Yaw threshold type"() -> (w165:refnum<vi>)
      n96 = control-ref of="Pitch threshold type"() -> (w164:refnum<vi>)
      n97 = control-ref of="Roll threshold type"() -> (w163:refnum<vi>)
      n98 = control-ref of="Z gyro threshold type"() -> (w162:refnum<vi>)
      n99 = control-ref of="Y gyro threshold type"() -> (w161:refnum<vi>)
      n100 = control-ref of="X gyro threshold type"() -> (w160:refnum<vi>)
      n101 = control-ref of="Z accel threshold type"() -> (w159:refnum<vi>)
      n102 = control-ref of="Y accel threshold type"() -> (w158:refnum<vi>)
      n103 = control-ref of="X accel threshold type"() -> (w157:refnum<vi>)
      n104 = Bundle By Name(cluster=T12 {"Yaw threshold type"=refnum, "Pitch threshold type"=refnum, "Roll threshold type"=refnum, "Z gyro threshold type"=refnum, "Y gyro threshold type"=refnum, "X gyro threshold type"=refnum, "Z accel threshold type"=refnum, "Y accel threshold type"=refnum, "X accel threshold type"=refnum, "Set all Motion detection type configurations"=refnum, "Get all Motion detection type configurations"=refnum, "Set yaw threshold type"=refnum, "Get yaw threshold type"=refnum, "Set pitch threshold type"=refnum, "Get pitch threshold type"=refnum, "Set roll threshold type"=refnum, "Get roll threshold type"=refnum, "Set Z gyroscope threshold type"=refnum, "Get Z gyroscope threshold type"=refnum, "Set Y gyroscope threshold type"=refnum, "Get Y gyroscope threshold type"=refnum, "Set X gyroscope threshold type"=refnum, "Get X gyroscope threshold type"=refnum, "Set Z accel threshold type"=refnum, "Get Z accel threshold type"=refnum, "Set Y accel threshold type"=refnum, "Get Y accel threshold type"=refnum, "Get X accel threshold type"=refnum, "Set X accel threshold type"=refnum}, "Yaw threshold type"=w165, "Pitch threshold type"=w164, "Roll threshold type"=w163, "Z gyro threshold type"=w162, "Y gyro threshold type"=w161, "X gyro threshold type"=w160, "Z accel threshold type"=w159, "Y accel threshold type"=w158, "X accel threshold type"=w157) -> (w156:T12)
      n105 = control-ref of="Set all Motion detection type configurations"() -> (w155:refnum<vi>)
      n106 = control-ref of="Get all Motion detection type configurations"() -> (w154:refnum<vi>)
      n107 = control-ref of="Set yaw threshold type"() -> (w153:refnum<vi>)
      n108 = control-ref of="Get yaw threshold type"() -> (w152:refnum<vi>)
      n109 = control-ref of="Set pitch threshold type"() -> (w151:refnum<vi>)
      n110 = control-ref of="Get pitch threshold type"() -> (w150:refnum<vi>)
      n111 = control-ref of="Set roll threshold type"() -> (w149:refnum<vi>)
      n112 = control-ref of="Get roll threshold type"() -> (w148:refnum<vi>)
      n113 = control-ref of="Set Z gyroscope threshold type"() -> (w147:refnum<vi>)
      n114 = control-ref of="Get Z gyroscope threshold type"() -> (w146:refnum<vi>)
      n115 = control-ref of="Set Y gyroscope threshold type"() -> (w145:refnum<vi>)
      n116 = control-ref of="Get Y gyroscope threshold type"() -> (w144:refnum<vi>)
      n117 = control-ref of="Set X gyroscope threshold type"() -> (w143:refnum<vi>)
      n118 = control-ref of="Get X gyroscope threshold type"() -> (w142:refnum<vi>)
      n119 = control-ref of="Set Z accel threshold type"() -> (w141:refnum<vi>)
      n120 = control-ref of="Get Z accel threshold type"() -> (w140:refnum<vi>)
      n121 = control-ref of="Set Y accel threshold type"() -> (w139:refnum<vi>)
      n122 = control-ref of="Get Y accel threshold type"() -> (w138:refnum<vi>)
      n123 = control-ref of="Get X accel threshold type"() -> (w137:refnum<vi>)
      n124 = control-ref of="Set X accel threshold type"() -> (w136:refnum<vi>)
      n125 = Bundle By Name(cluster=w156, "Set all Motion detection type configurations"=w155, "Get all Motion detection type configurations"=w154, "Set yaw threshold type"=w153, "Get yaw threshold type"=w152, "Set pitch threshold type"=w151, "Get pitch threshold type"=w150, "Set roll threshold type"=w149, "Get roll threshold type"=w148, "Set Z gyroscope threshold type"=w147, "Get Z gyroscope threshold type"=w146, "Set Y gyroscope threshold type"=w145, "Get Y gyroscope threshold type"=w144, "Set X gyroscope threshold type"=w143, "Get X gyroscope threshold type"=w142, "Set Z accel threshold type"=w141, "Get Z accel threshold type"=w140, "Set Y accel threshold type"=w139, "Get Y accel threshold type"=w138, "Get X accel threshold type"=w137, "Set X accel threshold type"=w136) -> (w132:T12)
    }
  }
  n126 = flat-sequence {
    tunnel: w31 -> [w232]
    tunnel: [w232] -> w30
    tunnel: w26 -> [w172]
    tunnel: [w172] -> w25
    tunnel: w22 -> [w171]
    tunnel: [w171] -> w21
    tunnel: w19 -> [w170]
    tunnel: [w170] -> w18
    tunnel: w17 -> [w169]
    tunnel: [w169] -> w16
    tunnel: [w168] -> w15
    frame #0 {
      # "Motion detection threshold values"
      n127 = control-ref of="Yaw threshold (U)"() -> (w230:refnum<vi>)
      n128 = control-ref of="Yaw threshold (L)"() -> (w229:refnum<vi>)
      n129 = control-ref of="Pitch threshold (U)"() -> (w228:refnum<vi>)
      n130 = control-ref of="Pitch. threshold (L)"() -> (w227:refnum<vi>)
      n131 = control-ref of="Roll threshold (U)"() -> (w226:refnum<vi>)
      n132 = control-ref of="Roll threshold (L)"() -> (w225:refnum<vi>)
      n133 = control-ref of="Z gyro. threshold (U)"() -> (w224:refnum<vi>)
      n134 = control-ref of="Z gyro. threshold (L)"() -> (w223:refnum<vi>)
      n135 = control-ref of="Y gyro. threshold (U)"() -> (w222:refnum<vi>)
      n136 = control-ref of="Y gyro. threshold (L)"() -> (w221:refnum<vi>)
      n137 = control-ref of="X gyro. threshold (U)"() -> (w220:refnum<vi>)
      n138 = control-ref of="X gyro. threshold (L)"() -> (w219:refnum<vi>)
      n139 = control-ref of="Z accel. threshold (U)"() -> (w218:refnum<vi>)
      n140 = control-ref of="Z accel. threshold (L)"() -> (w217:refnum<vi>)
      n141 = control-ref of="Y accel. threshold (U)"() -> (w216:refnum<vi>)
      n142 = control-ref of="Y accel. threshold (L)"() -> (w215:refnum<vi>)
      n143 = control-ref of="X accel. threshold (U)"() -> (w214:refnum<vi>)
      n144 = control-ref of="X accel. threshold (L)"() -> (w213:refnum<vi>)
      n145 = Bundle By Name(cluster=T11 {"Yaw threshold (U)"=refnum, "Yaw threshold (L)"=refnum, "Pitch threshold (U)"=refnum, "Pitch. threshold (L)"=refnum, "Roll threshold (U)"=refnum, "Roll threshold (L)"=refnum, "Z gyro. threshold (U)"=refnum, "Z gyro. threshold (L)"=refnum, "Y gyro. threshold (U)"=refnum, "Y gyro. threshold (L)"=refnum, "X gyro. threshold (U)"=refnum, "X gyro. threshold (L)"=refnum, "Z accel. threshold (U)"=refnum, "Z accel. threshold (L)"=refnum, "Y accel. threshold (U)"=refnum, "Y accel. threshold (L)"=refnum, "X accel. threshold (U)"=refnum, "X accel. threshold (L)"=refnum, "Set all Motion detection threshold configurations"=refnum, "Get yaw threshold (upper)"=refnum, "Get yaw threshold (lower)"=refnum, "Get pitch threshold (upper)"=refnum, "Get pitch threshold (lower)"=refnum, "Get roll threshold (upper)"=refnum, "Get roll threshold (lower)"=refnum, "Get Z gyro threshold (upper)"=refnum, "Get Z gyro threshold (lower)"=refnum, "Get Y gyro threshold (upper)"=refnum, "Get Y gyro threshold (lower)"=refnum, "Get X gyro threshold (upper)"=refnum, "Get X gyro threshold (lower)"=refnum, "Get Z accel threshold (upper)"=refnum, "Get Z accel threshold (lower)"=refnum, "Get Y accel threshold (upper)"=refnum, "Get Y accel threshold (lower)"=refnum, "Get X accel threshold (upper)"=refnum, "Get X accel threshold (lower)"=refnum, "Get all Motion detection threshold configurations"=refnum, "Set yaw threshold (upper)"=refnum, "Set yaw threshold (lower)"=refnum, "Set pitch threshold (upper)"=refnum, "Set pitch threshold (lower)"=refnum, "Set roll threshold (upper)"=refnum, "Set roll threshold (lower)"=refnum, "Set Z gyro threshold (upper)"=refnum, "Set Z gyro threshold (lower)"=refnum, "Set Y gyro threshold (upper)"=refnum, "Set Y gyro threshold (lower)"=refnum, "Set X gyro threshold (upper)"=refnum, "Set X gyro threshold (lower)"=refnum, "Set Z accel threshold (upper)"=refnum, "Set Z accel threshold (lower)"=refnum, "Set Y accel threshold (upper)"=refnum, "Set Y accel threshold (lower)"=refnum, "Set X accel threshold (upper)"=refnum, "Set X accel threshold (lower)"=refnum}, "Yaw threshold (U)"=w230, "Yaw threshold (L)"=w229, "Pitch threshold (U)"=w228, "Pitch. threshold (L)"=w227, "Roll threshold (U)"=w226, "Roll threshold (L)"=w225, "Z gyro. threshold (U)"=w224, "Z gyro. threshold (L)"=w223, "Y gyro. threshold (U)"=w222, "Y gyro. threshold (L)"=w221, "X gyro. threshold (U)"=w220, "X gyro. threshold (L)"=w219, "Z accel. threshold (U)"=w218, "Z accel. threshold (L)"=w217, "Y accel. threshold (U)"=w216, "Y accel. threshold (L)"=w215, "X accel. threshold (U)"=w214, "X accel. threshold (L)"=w213) -> (w212:T11)
      n146 = control-ref of="Set all Motion detection threshold configurations"() -> (w211:refnum<vi>)
      n147 = control-ref of="Get yaw threshold (upper)"() -> (w210:refnum<vi>)
      n148 = control-ref of="Get yaw threshold (lower)"() -> (w209:refnum<vi>)
      n149 = control-ref of="Get pitch threshold (upper)"() -> (w208:refnum<vi>)
      n150 = control-ref of="Get pitch threshold (lower)"() -> (w207:refnum<vi>)
      n151 = control-ref of="Get roll threshold (upper)"() -> (w206:refnum<vi>)
      n152 = control-ref of="Get roll threshold (lower)"() -> (w205:refnum<vi>)
      n153 = control-ref of="Get Z gyro threshold (upper)"() -> (w204:refnum<vi>)
      n154 = control-ref of="Get Z gyro threshold (lower)"() -> (w203:refnum<vi>)
      n155 = control-ref of="Get Y gyro threshold (upper)"() -> (w202:refnum<vi>)
      n156 = control-ref of="Get Y gyro threshold (lower)"() -> (w201:refnum<vi>)
      n157 = control-ref of="Get X gyro threshold (upper)"() -> (w200:refnum<vi>)
      n158 = control-ref of="Get X gyro threshold (lower)"() -> (w199:refnum<vi>)
      n159 = control-ref of="Get Z accel threshold (upper)"() -> (w198:refnum<vi>)
      n160 = control-ref of="Get Z accel threshold (lower)"() -> (w197:refnum<vi>)
      n161 = control-ref of="Get Y accel threshold (upper)"() -> (w196:refnum<vi>)
      n162 = control-ref of="Get Y accel threshold (lower)"() -> (w195:refnum<vi>)
      n163 = control-ref of="Get X accel threshold (upper)"() -> (w194:refnum<vi>)
      n164 = control-ref of="Get X accel threshold (lower)"() -> (w193:refnum<vi>)
      n165 = Bundle By Name(cluster=w212, "Set all Motion detection threshold configurations"=w211, "Get yaw threshold (upper)"=w210, "Get yaw threshold (lower)"=w209, "Get pitch threshold (upper)"=w208, "Get pitch threshold (lower)"=w207, "Get roll threshold (upper)"=w206, "Get roll threshold (lower)"=w205, "Get Z gyro threshold (upper)"=w204, "Get Z gyro threshold (lower)"=w203, "Get Y gyro threshold (upper)"=w202, "Get Y gyro threshold (lower)"=w201, "Get X gyro threshold (upper)"=w200, "Get X gyro threshold (lower)"=w199, "Get Z accel threshold (upper)"=w198, "Get Z accel threshold (lower)"=w197, "Get Y accel threshold (upper)"=w196, "Get Y accel threshold (lower)"=w195, "Get X accel threshold (upper)"=w194, "Get X accel threshold (lower)"=w193) -> (w192:T11)
      n166 = control-ref of="Get all Motion detection threshold configurations"() -> (w191:refnum<vi>)
      n167 = control-ref of="Set yaw threshold (upper)"() -> (w190:refnum<vi>)
      n168 = control-ref of="Set yaw threshold (lower)"() -> (w189:refnum<vi>)
      n169 = control-ref of="Set pitch threshold (upper)"() -> (w188:refnum<vi>)
      n170 = control-ref of="Set pitch threshold (lower)"() -> (w187:refnum<vi>)
      n171 = control-ref of="Set roll threshold (upper)"() -> (w186:refnum<vi>)
      n172 = control-ref of="Set roll threshold (lower)"() -> (w185:refnum<vi>)
      n173 = control-ref of="Set Z gyro threshold (upper)"() -> (w184:refnum<vi>)
      n174 = control-ref of="Set Z gyro threshold (lower)"() -> (w183:refnum<vi>)
      n175 = control-ref of="Set Y gyro threshold (upper)"() -> (w182:refnum<vi>)
      n176 = control-ref of="Set Y gyro threshold (lower)"() -> (w181:refnum<vi>)
      n177 = control-ref of="Set X gyro threshold (upper)"() -> (w180:refnum<vi>)
      n178 = control-ref of="Set X gyro threshold (lower)"() -> (w179:refnum<vi>)
      n179 = control-ref of="Set Z accel threshold (upper)"() -> (w178:refnum<vi>)
      n180 = control-ref of="Set Z accel threshold (lower)"() -> (w177:refnum<vi>)
      n181 = control-ref of="Set Y accel threshold (upper)"() -> (w176:refnum<vi>)
      n182 = control-ref of="Set Y accel threshold (lower)"() -> (w175:refnum<vi>)
      n183 = control-ref of="Set X accel threshold (upper)"() -> (w174:refnum<vi>)
      n184 = control-ref of="Set X accel threshold (lower)"() -> (w173:refnum<vi>)
      n185 = Bundle By Name(cluster=w192, "Get all Motion detection threshold configurations"=w191, "Set yaw threshold (upper)"=w190, "Set yaw threshold (lower)"=w189, "Set pitch threshold (upper)"=w188, "Set pitch threshold (lower)"=w187, "Set roll threshold (upper)"=w186, "Set roll threshold (lower)"=w185, "Set Z gyro threshold (upper)"=w184, "Set Z gyro threshold (lower)"=w183, "Set Y gyro threshold (upper)"=w182, "Set Y gyro threshold (lower)"=w181, "Set X gyro threshold (upper)"=w180, "Set X gyro threshold (lower)"=w179, "Set Z accel threshold (upper)"=w178, "Set Z accel threshold (lower)"=w177, "Set Y accel threshold (upper)"=w176, "Set Y accel threshold (lower)"=w175, "Set X accel threshold (upper)"=w174, "Set X accel threshold (lower)"=w173) -> (w168:T11)
    }
  }
  n186 = flat-sequence {
    tunnel: w30 -> [w246]
    tunnel: [w246] -> w7
    tunnel: w25 -> [w238]
    tunnel: [w238] -> w13
    tunnel: w21 -> [w237]
    tunnel: [w237] -> w12
    tunnel: w18 -> [w236]
    tunnel: [w236] -> w11
    tunnel: w16 -> [w235]
    tunnel: [w235] -> w10
    tunnel: w15 -> [w234]
    tunnel: [w234] -> w9
    tunnel: [w233] -> w8
    frame #0 {
      # "Motion Processing Complementary Filter Constants"
      n187 = control-ref of="Set pitch filter constant"() -> (w244:refnum<vi>)
      n188 = control-ref of="Get pitch filter constant"() -> (w243:refnum<vi>)
      n189 = control-ref of="Set roll filter constant"() -> (w242:refnum<vi>)
      n190 = control-ref of="Get roll filter constant"() -> (w241:refnum<vi>)
      n191 = control-ref of="Pitch filter constant"() -> (w240:refnum<vi>)
      n192 = control-ref of="Roll filter constant"() -> (w239:refnum<vi>)
      n193 = Bundle By Name(cluster=T10 {"Set pitch filter constant"=refnum, "Get pitch filter constant"=refnum, "Set roll filter constant"=refnum, "Get roll filter constant"=refnum, "Pitch filter constant"=refnum, "Roll filter constant"=refnum} ("MP_Comp_Filter_Constants_Reference"), "Set pitch filter constant"=w244, "Get pitch filter constant"=w243, "Set roll filter constant"=w242, "Get roll filter constant"=w241, "Pitch filter constant"=w240, "Roll filter constant"=w239) -> (w233:T10)
    }
  }
  n194 = Bundle By Name(cluster=T8 {"IMU_configuration_references"={"Get all IMU configurations"=refnum, "Set all IMU configurations"=refnum, "Get sampling frequency"=refnum, "Set sampling frequency"=refnum, "Get calibration point count"=refnum, "Set calibration point count"=refnum, "Get calibration interval"=refnum, "Set calibration interval"=refnum, "Get Gyroscope bandwidth"=refnum, "Set Gyroscope bandwidth"=refnum, "Get Gyroscope F.S. Value"=refnum, "Set Gyroscope F.S. Value"=refnum, "Get Accelerometer bandwidth"=refnum, "Set Accelerometer bandwidth"=refnum, "Get Accelerometer F.S. Value"=refnum, "Set Accelerometer F.S. Value"=refnum, "Sampling frequency (Hz)"=refnum, "Calibration point count"=refnum, "Calibration interval (ms)"=refnum, "IMU Gyroscope bandwidth"=refnum, "IMU Gyroscope F.S. value"=refnum, "IMU Accelerometer bandwidth"=refnum, "IMU Accelerometer F.S. value"=refnum}, "MP_Comp_Filter_Constants_References"={"Set pitch filter constant"=refnum, "Get pitch filter constant"=refnum, "Set roll filter constant"=refnum, "Get roll filter constant"=refnum, "Pitch filter constant"=refnum, "Roll filter constant"=refnum}, "MD_Threshold_References"={"Yaw threshold (U)"=refnum, "Yaw threshold (L)"=refnum, "Pitch threshold (U)"=refnum, "Pitch. threshold (L)"=refnum, "Roll threshold (U)"=refnum, "Roll threshold (L)"=refnum, "Z gyro. threshold (U)"=refnum, "Z gyro. threshold (L)"=refnum, "Y gyro. threshold (U)"=refnum, "Y gyro. threshold (L)"=refnum, "X gyro. threshold (U)"=refnum, "X gyro. threshold (L)"=refnum, "Z accel. threshold (U)"=refnum, "Z accel. threshold (L)"=refnum, "Y accel. threshold (U)"=refnum, "Y accel. threshold (L)"=refnum, "X accel. threshold (U)"=refnum, "X accel. threshold (L)"=refnum, "Set all Motion detection threshold configurations"=refnum, "Get yaw threshold (upper)"=refnum, "Get yaw threshold (lower)"=refnum, "Get pitch threshold (upper)"=refnum, "Get pitch threshold (lower)"=refnum, "Get roll threshold (upper)"=refnum, "Get roll threshold (lower)"=refnum, "Get Z gyro threshold (upper)"=refnum, "Get Z gyro threshold (lower)"=refnum, "Get Y gyro threshold (upper)"=refnum, "Get Y gyro threshold (lower)"=refnum, "Get X gyro threshold (upper)"=refnum, "Get X gyro threshold (lower)"=refnum, "Get Z accel threshold (upper)"=refnum, "Get Z accel threshold (lower)"=refnum, "Get Y accel threshold (upper)"=refnum, "Get Y accel threshold (lower)"=refnum, "Get X accel threshold (upper)"=refnum, "Get X accel threshold (lower)"=refnum, "Get all Motion detection threshold configurations"=refnum, "Set yaw threshold (upper)"=refnum, "Set yaw threshold (lower)"=refnum, "Set pitch threshold (upper)"=refnum, "Set pitch threshold (lower)"=refnum, "Set roll threshold (upper)"=refnum, "Set roll threshold (lower)"=refnum, "Set Z gyro threshold (upper)"=refnum, "Set Z gyro threshold (lower)"=refnum, "Set Y gyro threshold (upper)"=refnum, "Set Y gyro threshold (lower)"=refnum, "Set X gyro threshold (upper)"=refnum, "Set X gyro threshold (lower)"=refnum, "Set Z accel threshold (upper)"=refnum, "Set Z accel threshold (lower)"=refnum, "Set Y accel threshold (upper)"=refnum, "Set Y accel threshold (lower)"=refnum, "Set X accel threshold (upper)"=refnum, "Set X accel threshold (lower)"=refnum}, "MD_Type_References"={"Yaw threshold type"=refnum, "Pitch threshold type"=refnum, "Roll threshold type"=refnum, "Z gyro threshold type"=refnum, "Y gyro threshold type"=refnum, "X gyro threshold type"=refnum, "Z accel threshold type"=refnum, "Y accel threshold type"=refnum, "X accel threshold type"=refnum, "Set all Motion detection type configurations"=refnum, "Get all Motion detection type configurations"=refnum, "Set yaw threshold type"=refnum, "Get yaw threshold type"=refnum, "Set pitch threshold type"=refnum, "Get pitch threshold type"=refnum, "Set roll threshold type"=refnum, "Get roll threshold type"=refnum, "Set Z gyroscope threshold type"=refnum, "Get Z gyroscope threshold type"=refnum, "Set Y gyroscope threshold type"=refnum, "Get Y gyroscope threshold type"=refnum, "Set X gyroscope threshold type"=refnum, "Get X gyroscope threshold type"=refnum, "Set Z accel threshold type"=refnum, "Get Z accel threshold type"=refnum, "Set Y accel threshold type"=refnum, "Get Y accel threshold type"=refnum, "Get X accel threshold type"=refnum, "Set X accel threshold type"=refnum}, "LED_Configuration_References"={"Get all LED configurations"=refnum, "Set all LED configurations"=refnum, "Get LED3 configuration"=refnum, "Set LED3 configuration"=refnum, "Get LED2 configuration"=refnum, "Set LED2 configuration"=refnum, "Get LED1 configuration"=refnum, "Set LED1 configuration"=refnum, "LED3 Configuration"=refnum, "LED2 Configuration"=refnum, "LED1 Configuration"=refnum}, "Primary_references"={"3D View Image"=refnum, "Plot"=refnum, "Graph / 3D view tab control"=refnum, "MP Reset"=refnum, "Calibrate IMU"=refnum, "Plot Parameter List"=refnum, "Remove Parameter from Plot"=refnum, "Add Parameter to Plot"=refnum, "Parameter to monitor"=refnum, "Yaw motion detection output"=refnum, "Pitch motion detection output"=refnum, "Roll motion detection output"=refnum, "Z gyro motion detection output"=refnum, "Y gyro motion detection output"=refnum, "X gyro motion detection output"=refnum, "Z accel motion detection output"=refnum, "Y accel motion detection output"=refnum, "X accel motion detection output"=refnum, "Yaw angle (filter) (degrees)"=refnum, "Pitch angle (filter) (degrees)"=refnum, "Roll angle (filter) (degrees)"=refnum, "Yaw angle (gyro) (degrees)"=refnum, "Pitch angle (gyro) (degrees)"=refnum, "Roll angle (gyro) (degrees)"=refnum, "Yaw angle (accel) (degrees)"=refnum, "Pitch angle (accel) (degrees)"=refnum, "Roll angle (accel) (degrees)"=refnum, "Z gyroscope reading (DPS)"=refnum, "Y gyroscope reading (DPS)"=refnum, "X gyroscope reading (DPS)"=refnum, "Z accelerometer reading (G)"=refnum, "Y accelerometer reading (G)"=refnum, "X accelerometer reading (G)"=refnum, "Save all config."=refnum, "Write all config."=refnum, "Read all config."=refnum, "Tab Control"=refnum, "Baud Rate"=refnum, "COM Port"=refnum, "Time (ms)"=refnum, "Value (Units)"=refnum, "Exit Application"=refnum, "Connect Device"=refnum, "Progress Bar"=refnum, "Get Range & Offset"=refnum, "Range"=refnum, "Offset"=refnum, "Set Range & Offset"=refnum, "Parameter name"=refnum, "Plot time (ms)"=refnum, "Plot value"=refnum}, "MPU_Stick_Queues"={"UI Event Handler"=refnum, "3D View Updater"=refnum, "Plot Updater"=refnum, "Serial Port Reader"=refnum, "UI Indicators Updater"=refnum}, "ADCP"=refnum} ("MPU_Stick_Globals"), "IMU_configuration_references"=w13, "Primary_references"=w12, "LED_Configuration_References"=w11, "MD_Type_References"=w10, "MD_Threshold_References"=w9, "MP_Comp_Filter_Constants_References"=w8) -> (w6:T8)
  n195 = call "MPU_Stick_Main_Init.vi"("error in (no error)"=w7, "MPU_Stick_Globals In"=w6) -> ("error out"=w1:errorcluster, "MPU_Stick_Globals Out"=w2:T8)  [unwired: 8 in]
  n196 = disable-structure shown="Enabled" {
    disable-tunnel: w2 -> [w248 _]
    disable-tunnel: w1 -> [w247 _]
    frame Enabled {
      n197 = call "MPU_Stick_Read_Serial_Port.vi"("error in (no error)"=w247, "MPU_Stick_Globals"=w248) -> ()  [unwired: 10 in]
    }
    frame Disabled {
    }
  }
  n198 = disable-structure shown="Disabled" {
    disable-tunnel: w2 -> [w250 _]
    disable-tunnel: w1 -> [w249 _]
    frame Disabled {
      n199 = call "MPU_Stick_Serial_Port_Emulator.vi"("error in (no error)"=w249, "MPU_Stick_Globals"=w250) -> ()  [unwired: 10 in]
    }
    frame Enabled {
    }
  }
  n200 = disable-structure shown="Enabled" {
    disable-tunnel: w2 -> [w252 _]
    disable-tunnel: w1 -> [w251 _]
    frame Enabled {
      n201 = call "MPU_Stick_Plot_Updater.vi"("error in (no error)"=w251, "MPU_Stick_Globals"=w252) -> ()  [unwired: 10 in]
    }
    frame Disabled {
    }
  }
  n202 = call "MPU_Stick_UI_Event_Handler.vi"("error in (no error)"=w1, "MPU_Stick_Globals"=w2) -> ()  [unwired: 10 in]
  n203 = call "MPU_Stick_UI_Indicators_Updator.vi"("error in (no error)"=w1, "MPU_Stick_Globals"=w2) -> ()  [unwired: 10 in]
  n204 = call "MPU_Stick_3D_View_Updater.vi"("error in (no error)"=w1, "MPU_Stick_Globals"=w2) -> ()  [unwired: 10 in]
